vi "Set Motor ON ESP.vi"(8 "error in (no error)":errorcluster, 9 "Axis (1)":i32=1 min=1 max=3, 10 "VISA resource name":refnum<visa-resource-name>, 11 "ESP301 in":refnum<class "ESP301.lvclass">) -> (0 "error out":errorcluster, 2 "VISA resource name out":refnum<visa-resource-name>, 3 "ESP301 out":refnum<class "ESP301.lvclass">)   [LabVIEW 2020, in "ESP301.lvclass"]
uses:
  ESP301.lvclass
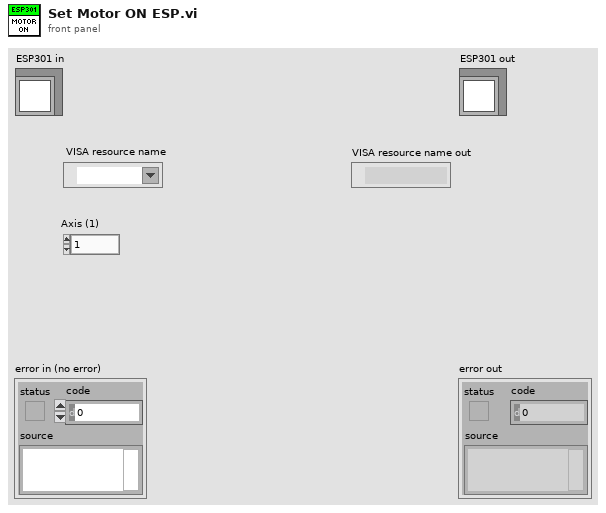
[diagram p1: front panel]
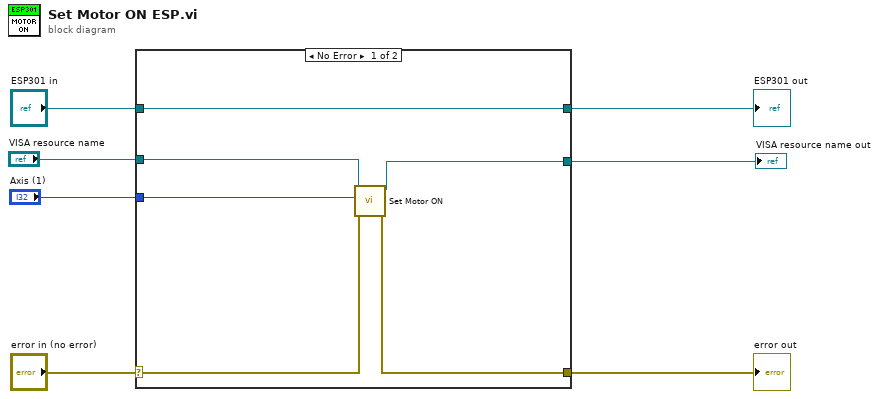
[diagram p0: block diagram]
diagram:
  n1 = case shown="No Error" "error in (no error)" {
    selector: "error in (no error)" -> [w9 w16]
    tunnel: [w8 w16] -> w6
    tunnel: [w13 w15] -> w4
    tunnel: "ESP301 in" -> [w13 w15]
    tunnel: "VISA resource name" -> [w12 w14]
    tunnel: "Axis (1)" -> [w11 _]
    tunnel: [w10 w14] -> w1
    frame No Error {
      n2 = call "Set Motor ON.vi"("error in (no error)"=w9, "Axis (1)"=w11, "VISA resource name"=w12) -> ("error out"=w8:errorcluster, "VISA resource name out"=w10:refnum<visa-resource-name>)  [unwired: 3 in]
    }
    frame Error {
    }
  }
  "error out" <- w6
  "ESP301 out" <- w4
  "VISA resource name out" <- w1
